vi "Write Single Device.vi"(6 "Index":i32, 7 "Section":string, 8 "error in (no error)":errorcluster, 10 "Device":refnum<class "Device.lvclass">, 11 "refnum":T1) -> (0 "error out":errorcluster, 3 "refnum out":T1)   [LabVIEW 2020, in "PicoG-App.lvlib" / "App.lvclass"]
uses:
  App.lvclass
  Device/Device.lvclass
  <vilib>/Utility/config.llb/NI_LVConfig.lvlib
  <vilib>/Utility/config.llb/Write Key (String).vi
  Builds/picoG/ppl/PicoG-Core.lvlibp/PicoG-Processor/PicoG-Core/DeployResource/DeployResource.lvclass
  <vilib>/Utility/config.llb/Config Data RefNum.ctl
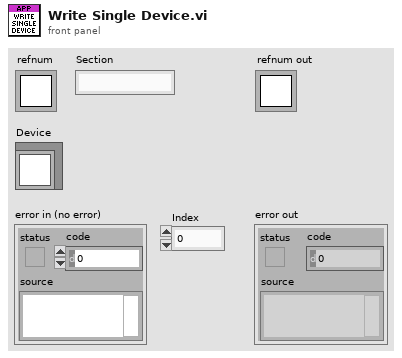
[diagram p1: front panel]
types:
  T1 = typedef "NI_LVConfig.lvlib/Config Data RefNum.ctl" = refnum<k1>
  T2 = typedef "PicoG-Core.lvlibp/DeployResource.lvclass/Config Item.ctl" = cluster{"Key":string, "Value":string}
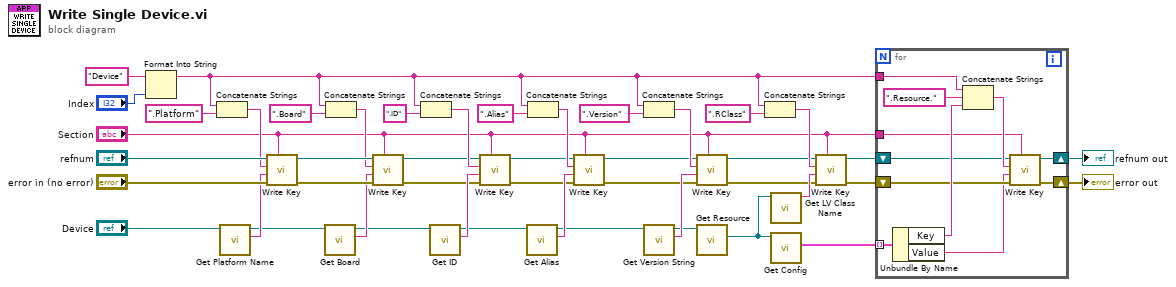
[diagram p0: block diagram]
diagram:
  n1 = Format Into String(initial string="Device", "Index") -> (resulting string=w4:string)  [unwired: 2 in, 1 out]
  n2 = Concatenate Strings(w4, ".Platform" ("string")) -> (w35:string)
  n3 = call "Get Platform Name.vi"("Device in"="Device") -> ("Platform"=w34:string, "Device out"=w33:refnum<class "Device.lvclass">)  [unwired: 8 in, 1 out]
  n4 = call-poly <vilib>:"Write Key.vi"("section"="Section", "error in (no error)"="error in (no error)", "value"=w34, "key"=w35, "refnum"="refnum") -> ("error out"=w31:errorcluster, "refnum out"=w32:T1)  [unwired: 4 in, 1 out]
  n5 = call "Get Board.vi"("Device in"=w33) -> ("Board"=w29:string, "Device out"=w28:refnum<class "Device.lvclass">)  [unwired: 8 in, 1 out]
  n6 = Concatenate Strings(w4, ".Board" ("string")) -> (w30:string)
  n7 = call-poly <vilib>:"Write Key.vi"("section"="Section", "error in (no error)"=w31, "value"=w29, "key"=w30, "refnum"=w32) -> ("error out"=w24:errorcluster, "refnum out"=w25:T1)  [unwired: 4 in, 1 out]
  n8 = Concatenate Strings(w4, ".ID" ("string")) -> (w26:string)
  n9 = call "Get ID.vi"("Device in"=w28) -> ("Id"=w27:string, "Device out"=w22:refnum<class "Device.lvclass">)  [unwired: 8 in, 1 out]
  n10 = call-poly <vilib>:"Write Key.vi"("section"="Section", "error in (no error)"=w24, "value"=w27, "key"=w26, "refnum"=w25) -> ("error out"=w19:errorcluster, "refnum out"=w20:T1)  [unwired: 4 in, 1 out]
  n11 = call "Get Alias.vi"("Device in"=w22) -> ("Alias"=w21:string, "Device out"=w17:refnum<class "Device.lvclass">)  [unwired: 8 in, 1 out]
  n12 = Concatenate Strings(w4, ".Alias" ("string")) -> (w23:string)
  n13 = call-poly <vilib>:"Write Key.vi"("section"="Section", "error in (no error)"=w19, "value"=w21, "key"=w23, "refnum"=w20) -> ("error out"=w14:errorcluster, "refnum out"=w15:T1)  [unwired: 4 in, 1 out]
  n14 = Concatenate Strings(w4, ".Version" ("string")) -> (w18:string)
  n15 = call "Get Version String.vi"("Device in"=w17) -> ("Version"=w16:string, "Device out"=w13:refnum<class "Device.lvclass">)  [unwired: 8 in, 1 out]
  n16 = call-poly <vilib>:"Write Key.vi"("section"="Section", "error in (no error)"=w14, "value"=w16, "key"=w18, "refnum"=w15) -> ("error out"=w9:errorcluster, "refnum out"=w10:T1)  [unwired: 4 in, 1 out]
  n17 = call "Get Resource.vi"("Device in"=w13) -> ("Resource"=w8:refnum<class "DeployResource.lvclass">)  [unwired: 8 in, 2 out]
  n18 = Concatenate Strings(w4, ".RClass" ("string")) -> (w12:string)
  n19 = call <vilib>:"Get LV Class Name.vi"("object"=w8) -> ("class name"=w11:string)  [unwired: 9 in, 1 out]
  n20 = call-dynamic "Get Config.vi"("DeployResource in"=w8) -> ("Config"=w5:T2[])  [unwired: 8 in, 2 out]
  n21 = call-poly <vilib>:"Write Key.vi"("section"="Section", "error in (no error)"=w9, "value"=w11, "key"=w12, "refnum"=w10) -> ("error out"=w6:errorcluster, "refnum out"=w7:T1)  [unwired: 4 in, 1 out]
  n22 = for {
    shift-right: [w47] -> w2
    shift-left: w7 -> [w51]
    shift-right: [w48] -> w1
    shift-left: w6 -> [w50]
    tunnel: w5 -> [w55] mode=indexing
    tunnel: w4 -> [w56]
    tunnel: "Section" -> [w52]
    n23 = Unbundle By Name(w55) -> ("Key"=w54:string, "Value"=w49:string)
    n24 = Concatenate Strings(w56, ".Resource." ("string"), w54) -> (w53:string)
    n25 = call-poly <vilib>:"Write Key.vi"("section"=w52, "error in (no error)"=w50, "value"=w49, "key"=w53, "refnum"=w51) -> ("error out"=w48:errorcluster, "refnum out"=w47:T1)  [unwired: 4 in, 1 out]
  }
  "error out" <- w1
  "refnum out" <- w2
